vi "Clear-object.vi"(8 "error in (no error)":errorcluster, 11 "Reference in":T1) -> (0 "error out":errorcluster, 3 "Reference out":T1)   [LabVIEW 2013, in "Server.lvlib" / "Server.lvclass"]
uses:
  Server.lvclass
  Object-reference.ctl
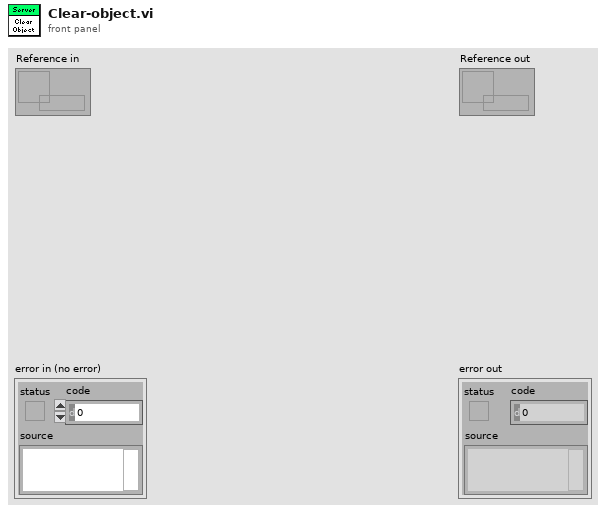
[diagram p1: front panel]
types:
  T1 = typedef "Server.lvlib/Server.lvclass/Object-reference.ctl" = refnum<data-value>
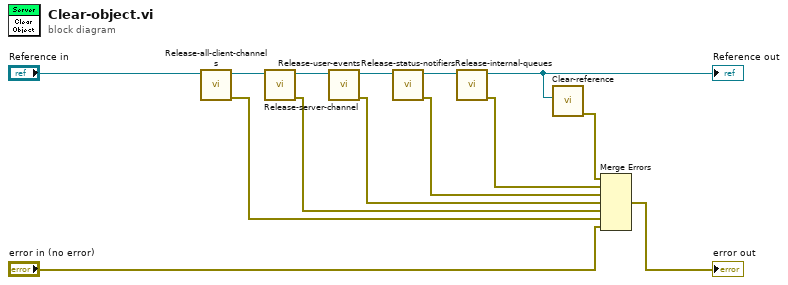
[diagram p0: block diagram]
diagram:
  n1 = call "Release-all-client-channels.vi"("ModComm in"="Reference in") -> ("error out"=w8:errorcluster, "ModComm out"=w12:T1)  [unwired: 9 in]
  n2 = call "Release-server-channel.vi"("ModComm in"=w12) -> ("error out"=w7:errorcluster, "ModComm out"=w11:T1)  [unwired: 9 in]
  n3 = call "Release-user-events.vi"("ModComm in"=w11) -> ("error out"=w6:errorcluster, "ModComm out"=w10:T1)  [unwired: 9 in]
  n4 = call "Release-status-notifiers.vi"("ModComm in"=w10) -> ("error out"=w5:errorcluster, "ModComm out"=w9:T1)  [unwired: 9 in]
  n5 = call "Release-internal-queues.vi"("ModComm in"=w9) -> ("error out"=w4:errorcluster, "ModComm out"=w13:T1)  [unwired: 9 in]
  "Reference out" <- w13
  n6 = call "Clear-reference.vi"("Object reference"=w13) -> ("error out"=w3:errorcluster)  [unwired: 9 in, 1 out]
  n7 = Merge Errors(w3, w4, w5, w6, w7, w8, "error in (no error)") -> (→"error out":errorcluster)
